vi "limitSwitchGlobals.vi"() -> ()   [LabVIEW 2014]
panel:
  out "bottomLimit":bool
  out "topLimit":bool
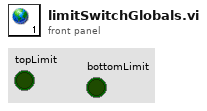
[diagram p1: front panel]
diagram:
